vi "Change plot.vi"(11 "XYGraph Ref In":refnum<vi>) -> ()   [LabVIEW 2017, in "DTacq Plot Display Library.lvlib"]
uses:
  DTacq Plot Display Library.lvlib
  Typedefs/Plot Channel Configruation--Cluster.ctl
panel:
  in  "Active Tab":u32
  in  "Page Configurations In":T2(array[cluster])
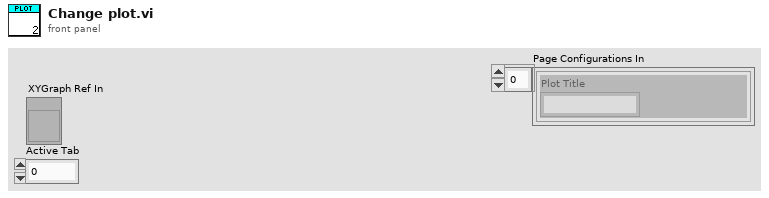
[diagram p1: front panel]
types:
  T1 = typedef "DTacq Plot Display Library.lvlib/Plot Channel Configruation--Cluster.ctl" = cluster{"Shared Variable Reference":refnum<k21>, "Full Variable Name":string, "URL":string, "Descriptive Name":string, "Data Type":variant, "Colour":u32}
  T2 = cluster{"Plot Title":string, "Y-Axis Label":string, "X-Axis Label":string, "Plot Channel Configurations":T1[]}[]
  T3 = cluster{"Plot Title":string, "Y-Axis Label":string, "X-Axis Label":string, "Plot Channel Configurations":T1[]}
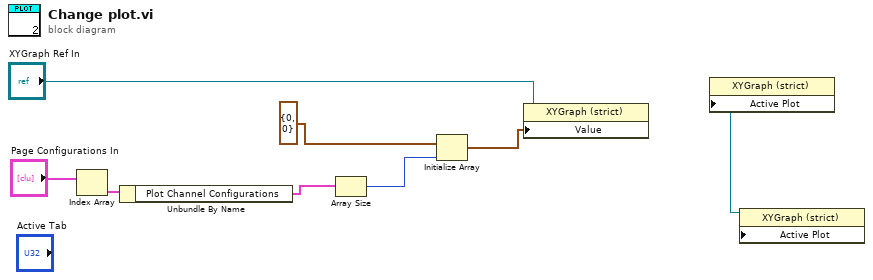
[diagram p0: block diagram]
diagram:
  n1 = Index Array(array="Page Configurations In") -> (element=w6:T3)  [unwired: 1 in]
  n2 = Unbundle By Name(w6) -> ("Plot Channel Configurations"=w5:T1[])
  n3 = Array Size(array=w5) -> (size(s)=w2:i32)
  n4 = Initialize Array(cluster{"X":i16, "Y":i16} {"X"=0, "Y"=0}, w2) -> (w1:cluster{"X":i16, "Y":i16}[])
  n5 = property class="XYGraph (strict)"(reference="XYGraph Ref In", "Value"=w1) -> ()  [unwired: 1 in, 2 out]
  n6 = property class="XYGraph (strict)" props=["Active Plot"]() -> (reference=w7:refnum<vi>)  [unwired: 2 in, 2 out]
  n7 = property class="XYGraph (strict)" props=["Active Plot"](reference=w7) -> ()  [unwired: 2 in, 2 out]
